vi "Haptic Master UDP.vi"() -> ()   [LabVIEW 2013]
uses:
  Common/controls/Vector3D Fingers.ctl
  labview_ros/omni_msgs/OmniFeedback.ctl
  labview_ros/geometry_msgs/Vector3.ctl
  Common/classes/MF3/MF3.lvclass
  <vilib>/Platform/TimedLoop/XDataNode/timing_clust.ctl
  <vilib>/Platform/TimedLoop/XDataNode/nitl_modes.ctl
  <vilib>/Platform/TimedLoop/XDataNode/wakeup.ctl
  labview_ros/geometry_msgs/Pose.ctl
  labview_ros/geometry_msgs/Point.ctl
  labview_ros/geometry_msgs/Quaternion.ctl
  labview_ros/omni_msgs/OmniState.ctl
  labview_ros/std_msgs/Header.ctl
  <userlib>/_matio/level5/Public/Write/Append Data Element.llb/Append Data Element (1D Array of Double).vi
  <userlib>/_matio/level5/Public/Write/Append Data Element.llb/Append Data Element (2D Array of Double).vi
  <vilib>/Platform/TimedLoop/XDataNode/XDataNode.xnode
  <userlib>/_matio/level5.lvlib
  <vilib>/Platform/TimedLoop/XDataNode/XDNodeRunTimeDep.lvlib
panel:
  out "OmniFeedback":T1
  out "Finger Positions":T3
  out "UDP Receiver":cluster{"Rate (Hz)":dbl, "Status":errorcluster}
  out "UDP Sender":cluster{"Rate (Hz)":dbl, "Status":errorcluster}
  in  "ROS Machine":T4={"IP"="192.168.0.10", "Read Port"=5053, "Write Port"=5054}
  in  "MasterFinger":T5={"PID Gains"={"Proportional Gain"=20, "Integral Gain"=5, "Derivative Gain"=0}, "Current limit"=0.0} {"Current limit" min=0.0 max=1.0 step=0.1}
  in  "Data Logging":cluster{"Path":path, "Save":bool}={"Path"=path "c:/ni-rt/testing/haptic_master.mat", "Save"=FALSE}
  out "Logging Status":errorcluster
  out "MasterFinger Status":errorcluster
  in  "Stop":bool
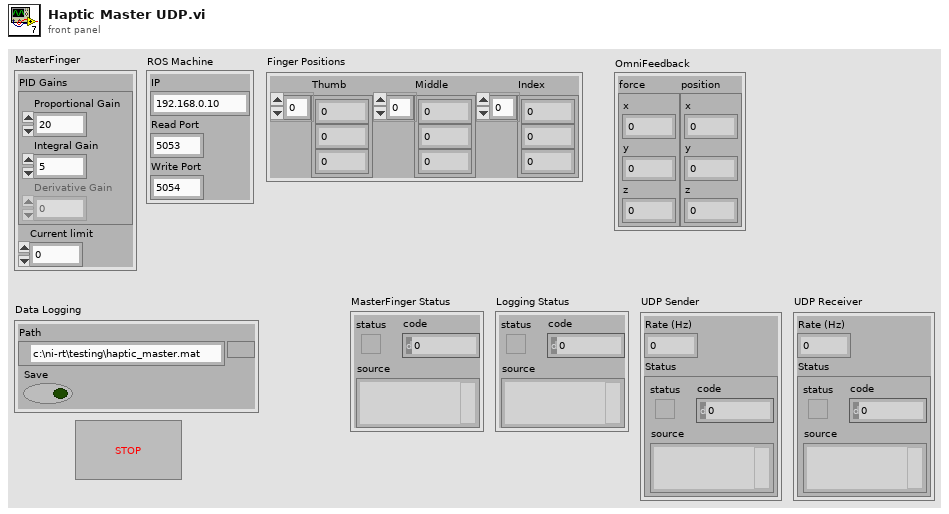
[diagram p1: front panel]
types:
  T1 = typedef "OmniFeedback.ctl" = cluster{"force":T2, "position":T2}
  T2 = typedef "Vector3.ctl" = cluster{"x":dbl, "y":dbl, "z":dbl}
  T3 = typedef "Vector3D Fingers.ctl" = cluster{"Thumb":dbl[], "Middle":dbl[], "Index":dbl[]}
  T4 = cluster{"IP":string, "Read Port":u16, "Write Port":u16}
  T5 = cluster{"PID Gains":cluster{"Proportional Gain":i16, "Integral Gain":i16, "Derivative Gain":i16}, "Current limit":dbl}
  T6 = typedef "Pose.ctl" = cluster{"position":T7, "orientation":T8}
  T7 = typedef "Point.ctl" = cluster{"x":dbl, "y":dbl, "z":dbl}
  T8 = typedef "Quaternion.ctl" = cluster{"x":dbl, "y":dbl, "z":dbl, "w":dbl}
  T9 = cluster{"Proportional Gain":i16, "Integral Gain":i16, "Derivative Gain":i16}
  T10 = typedef "XDNodeRunTimeDep.lvlib/timing_clust.ctl" = cluster{"Expected End [f-1]":u64, "Actual End [f-1]":u64, "Finished Late? [f-1]":bool, "Expected End [i-1]":u64, "Actual End [i-1]":u64, "Finished Late? [i-1]":bool, "Expected Start [i]":u64, "Actual Start [i]":u64, "Expected Start [f]":u64, "Actual Start [f]":u64, "Source Name":string, "Structure Name":string, "Period":i64, "Deadline":i64, "Offset":i64, "Start":i64, "Priority":i32, "Timeout":i32, "Mode":T11, "Wakeup Reason":T12, "Error":errorcluster, "Source Type":string, "Secondary Source Type":string, "Global End Time":u64, "Global Start Time":u64, "Frame Duration":u64, "Iteration Duration":u64, "Assigned CPU":i32, "I/O Scan Engine Mode":u32}
  T11 = typedef "XDNodeRunTimeDep.lvlib/nitl_modes.ctl" = enum32{"No Change", "Process missed periods, maintain original phase", "Discard missed periods, maintain original phase", "Process missed periods, ignore original phase", "Discard missed periods, ignore original phase"}
  T12 = typedef "XDNodeRunTimeDep.lvlib/wakeup.ctl" = enum32{"Normal", "Aborted", "Asynchronous wakeup", "Timing source error", "Timed loop error", "Timeout"}
  T13 = enum16{"big-endian, network order", "native, host order", "little-endian"}
  T14 = typedef "OmniState.ctl" = cluster{"header":T15, "locked":bool, "close_gripper":bool, "pose":T6, "current":T2, "velocity":T2}
  T15 = typedef "Header.ctl" = cluster{"seq":u32, "stamp":cluster{"sec":i32, "nsec":i32}, "frame_id":string}
  T16 = enum16{"open", "replace", "create", "open or create", "replace or create", "replace or create with confirmation"}
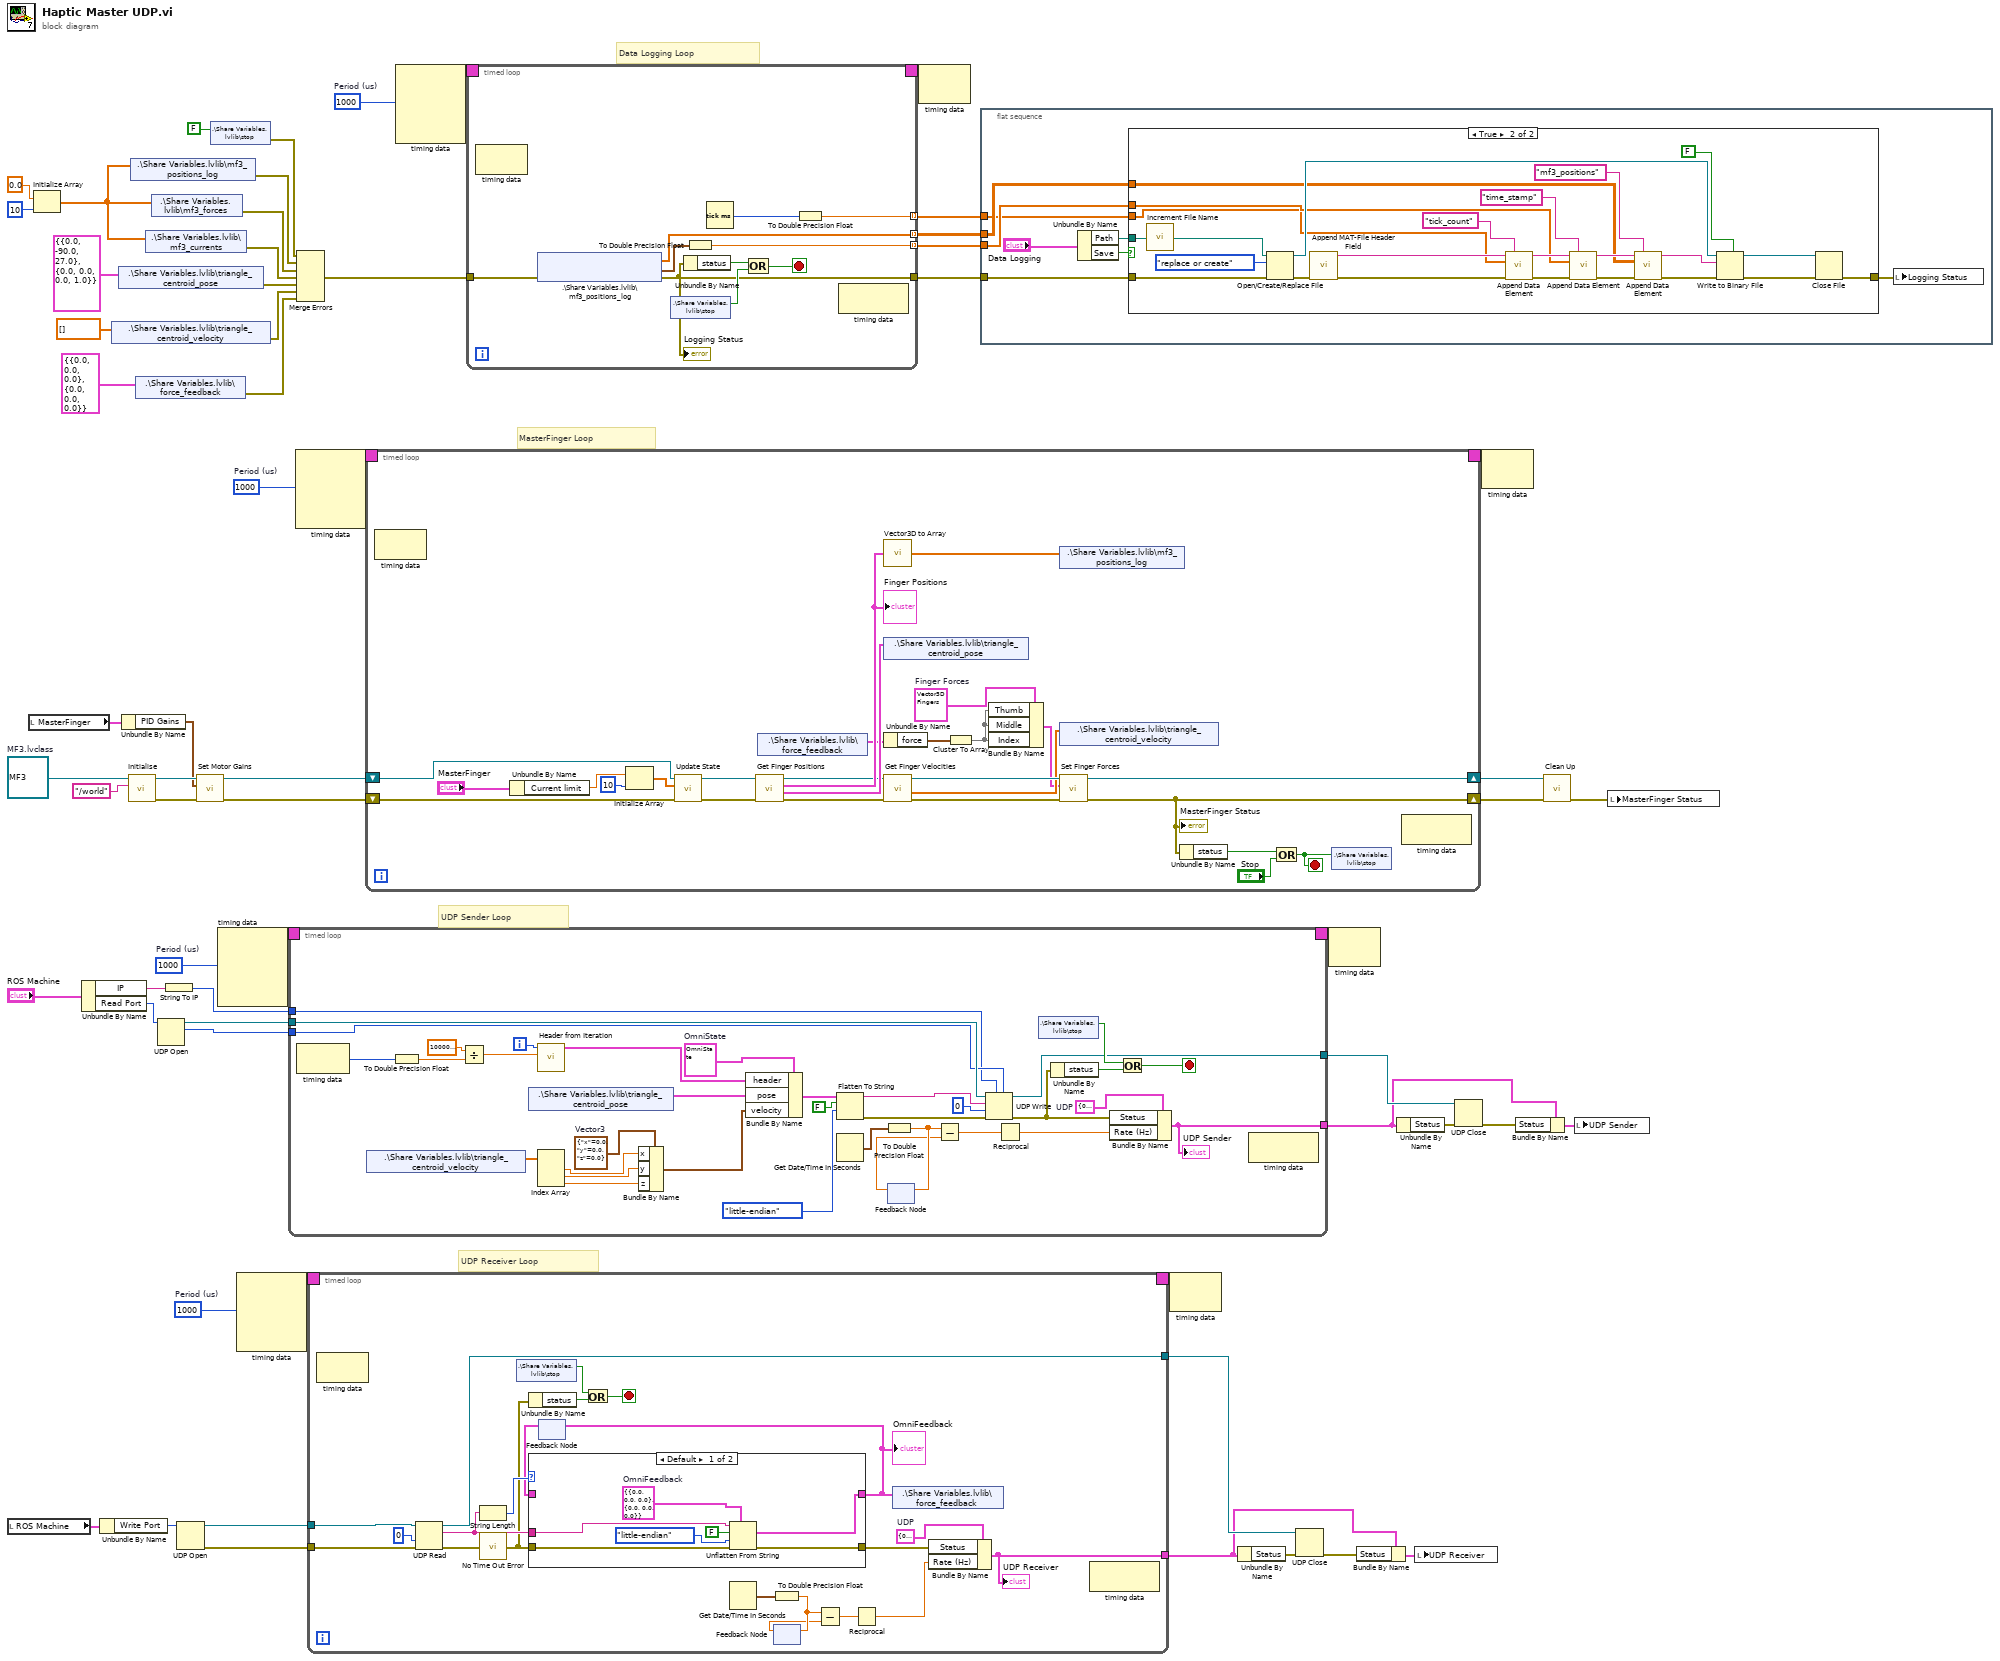
[diagram p0: block diagram]
diagram:
  w27 = i64 1000  # Period (us)
  w30 = i64 1000  # Period (us)
  w33 = i64 1000  # Period (us)
  w34 = i64 1000  # Period (us)
  w62 = refnum<class "MF3.lvclass"> refnum  # MF3.lvclass
  # "UDP Receiver Loop"
  # "UDP Sender Loop"
  # "Data Logging Loop"
  # "MasterFinger Loop"
  n1 = local read "ROS Machine"() -> (w23:T4)
  n2 = local read "MasterFinger"() -> (w44:T5)
  n3 = Initialize Array "Initialize Array"(0.0 ("element"), 10 ("dimension size")) -> (w41:dbl[])
  n4 = Unbundle By Name("ROS Machine") -> ("IP"=w26:string, "Read Port"=w24:u16)
  n5 = Unbundle By Name(w23) -> ("Write Port"=w22:u16)
  n6 = shared-variable ".\\Share Variables.lvlib\\triangle_centroid_velocity"(dbl[] [] ("triangle_centroid_velocity")) -> (error out=w4:errorcluster)  [unwired: 1 in]
  n7 = shared-variable ".\\Share Variables.lvlib\\triangle_centroid_pose"(T6 {"position"={"x"=0.0, "y"=-90.0, "z"=27.0}, "orientation"={"x"=0.0, "y"=0.0, "z"=0.0, "w"=1.0}} ("triangle_centroid_pose")) -> (error out=w6:errorcluster)  [unwired: 1 in]
  n8 = Unbundle By Name(w44) -> ("PID Gains"=w43:T9)
  n9 = call "Initialise.vi"("frame"="/world", "MF3 in"=w62) -> ("error out"=w45:errorcluster, "MF3 out"=w46:refnum<class "MF3.lvclass">)  [unwired: 8 in]
  n10 = shared-variable ".\\Share Variables.lvlib\\mf3_positions_log"(w41) -> (error out=w57:errorcluster)  [unwired: 1 in]
  n11 = shared-variable ".\\Share Variables.lvlib\\force_feedback"(T1 {"force"={"x"=0.0, "y"=0.0, "z"=0.0}, "position"={"x"=0.0, "y"=0.0, "z"=0.0}} ("force_feedback")) -> (error out=w1:errorcluster)  [unwired: 1 in]
  n12 = shared-variable ".\\Share Variables.lvlib\\mf3_currents"(w41) -> (error out=w55:errorcluster)  [unwired: 1 in]
  n13 = shared-variable ".\\Share Variables.lvlib\\mf3_forces"(w41) -> (error out=w56:errorcluster)  [unwired: 1 in]
  n14 = UDP Open(11:w24) -> (port=w21:refnum<k16>, 2:w20:u16)  [unwired: 1 in, 4 out]
  n15 = String To IP(1:w26) -> (0:w19:u32)
  n16 = UDP Open(11:w22) -> (port=w10:refnum<k16>, 0:w13:errorcluster)  [unwired: 1 in, 4 out]
  n17 = call "Set Motor Gains.vi"("error in (no error)"=w45, "motor gains"=w43, "MF3 in"=w46) -> ("error out"=w35:errorcluster, "MF3 out"=w36:refnum<class "MF3.lvclass">)  [unwired: 7 in]
  n18 = shared-variable ".\\Share Variables.lvlib\\stop"(FALSE ("stop")) -> (error out=w58:errorcluster)  [unwired: 1 in]
  n19 = node-c288(w30) -> (w32:T10)  [unwired: 3 in]
  n20 = node-c288(w27) -> (w29:T10)  [unwired: 3 in]
  n21 = timed-loop {
    timing: w32 -> [_]
    timing-out: [_] -> w31
    tunnel: w21 -> [w88]
    tunnel: w20 -> [w87]
    tunnel: w19 -> [w86]
    tunnel: [w76] -> w18
    tunnel: [w74] -> w15
    i -> [w77]
    stop <- w81 stop-if-true
    w73 = T2 {"x"=0.0, "y"=0.0, "z"=0.0}  # Vector3
    w80 = T14 {"header"={"seq"=0, "stamp"={"sec"=0, "nsec"=0}, "frame_id"=""}, "locked"=FALSE, "close_gripper"=FALSE, "pose"={"position"={"x"=0.0, "y"=0.0, "z"=0.0}, "orientation"={"x"=0.0, "y"=0.0, "z"=0.0, "w"=0.0}}, "current"={"x"=0.0, "y"=0.0, "z"=0.0}, "velocity"={"x"=0.0, "y"=0.0, "z"=0.0}}  # OmniState
    w75 = cluster{"Rate (Hz)":dbl, "Status":errorcluster} {"Rate (Hz)"=0.0, "Status"={"status"=FALSE, "code"=0, "source"=""}}  # UDP
    n22 = node-c288() -> (w66:i64)  [unwired: 1 in]
    n23 = shared-variable ".\\Share Variables.lvlib\\triangle_centroid_velocity"() -> (w72:dbl[])  [unwired: 1 in, 1 out]
    n24 = To Double Precision Float(number=w66) -> (double precision float=w65:dbl)
    n25 = Divide(x=1000000.0, y=w65) -> (x/y=w63:dbl)
    n26 = shared-variable ".\\Share Variables.lvlib\\triangle_centroid_pose"() -> (w67:T6)  [unwired: 1 in, 1 out]
    n27 = call "Header from Iteration.vi"("Rate (Hz)"=w63, "Iteration"=w77) -> ("Header"=w78:T15)  [unwired: 9 in]
    n28 = Index Array(array=w72) -> (element #1=w71:dbl, element #2=w70:dbl, element #3=w69:dbl)  [unwired: 3 in]
    n29 = Bundle By Name(cluster=w73, "x"=w71, "y"=w70, "z"=w69) -> (w68:T2)
    n30 = Bundle By Name(cluster=w80, "header"=w78, "pose"=w67, "velocity"=w68) -> (w79:T14)
    n31 = Flatten To String(anything=w79, prepend array or string size? (T)=FALSE, byte order (0:big-endian, network order)=T13."little-endian") -> (data string=w89:string, error out=w85:errorcluster)  [unwired: 1 in, 1 out]
    n32 = Get Date/Time In Seconds() -> (seconds since 1Jan1904=w94:timestamp)
    n33 = To Double Precision Float(number=w94) -> (double precision float=w92:dbl)
    n34 = feedback #1() -> (w91:dbl)  [unwired: 1 in]
    n35 = feedback-in #1(w92) -> ()
    n36 = Subtract(x=w92, y=w91) -> (x-y=w95:dbl)
    n37 = UDP Write(address=w86, port or service name=w87, connection ID=w88, data in=w89, 8:w85, 9:0 ("timeout ms (25000)")) -> (error out=w84:errorcluster, 3:w76:refnum<k16>)
    n38 = Reciprocal(x=w95) -> (1/x=w93:dbl)
    n39 = shared-variable ".\\Share Variables.lvlib\\stop"() -> (w83:bool)  [unwired: 1 in, 1 out]
    n40 = Unbundle By Name(w84) -> ("status"=w82:bool)
    n41 = Bundle By Name(cluster=w75, "Status"=w84, "Rate (Hz)"=w93) -> (w74:cluster{"Rate (Hz)":dbl, "Status":errorcluster})
    "UDP Sender" <- w74
    n42 = Or(x=w83, y=w82) -> (x .or. y?=w81:bool)
    n43 = node-c288() -> ()  [unwired: 1 in, 1 out]
  }
  n44 = node-c288(w34) -> (w40:T10)  [unwired: 3 in]
  n45 = Merge Errors(w58, w57, w56, w55, w6, w4, w1) -> (w48:errorcluster)
  n46 = timed-loop {
    timing: w29 -> [_]
    timing-out: [_] -> w28
    tunnel: w13 -> [w112]
    tunnel: w10 -> [w111]
    tunnel: [w110] -> w9
    tunnel: [w115] -> w8
    stop <- w107 stop-if-true
    w116 = cluster{"Rate (Hz)":dbl, "Status":errorcluster} {"Rate (Hz)"=0.0, "Status"={"status"=FALSE, "code"=0, "source"=""}}  # UDP
    n47 = node-c288() -> ()  [unwired: 1 in, 1 out]
    n48 = UDP Read(connection ID=w111, timeout ms (25000)=0 ("timeout (ms)"), 8:w112) -> (data out=w105:string, error out=w114:errorcluster, 3:w110:refnum<k16>)  [unwired: 1 in, 2 out]
    n49 = String Length(string=w105) -> (length=w106:i32)
    n50 = call <vilib>:"No Time Out Error.vi"("error in (no error)"=w114) -> ("error out"=w104:errorcluster)  [unwired: 14 out]
    n51 = shared-variable ".\\Share Variables.lvlib\\stop"() -> (w108:bool)  [unwired: 1 in, 1 out]
    n52 = Unbundle By Name(w104) -> ("status"=w109:bool)
    n53 = feedback #2() -> (w103:T1)  [unwired: 1 in]
    n54 = case shown="Default" w106 {
      tunnel: w104 -> [w123 w130]
      tunnel: [w127 w130] -> w102
      tunnel: [w125 w129] -> w101
      tunnel: w105 -> [w124 _]
      tunnel: w103 -> [_ w129]
      frame Default {
        w122 = T1 {"force"={"x"=0.0, "y"=0.0, "z"=0.0}, "position"={"x"=0.0, "y"=0.0, "z"=0.0}}  # OmniFeedback
        n55 = Unflatten From String(type=w122, binary string=w124, data includes array or string size? (T)=FALSE, byte order (0:big-endian, network order)=T13."little-endian", error in (no error)=w123) -> (value=w125:T1, error out=w127:errorcluster)  [unwired: 1 out]
      }
      frame 0 {
      }
    }
    "OmniFeedback" <- w101
    n56 = feedback-in #2(w101) -> ()
    n57 = Or(x=w108, y=w109) -> (x .or. y?=w107:bool)
    n58 = Get Date/Time In Seconds() -> (seconds since 1Jan1904=w120:timestamp)
    n59 = To Double Precision Float(number=w120) -> (double precision float=w118:dbl)
    n60 = feedback #3() -> (w117:dbl)  [unwired: 1 in]
    n61 = feedback-in #3(w118) -> ()
    n62 = Subtract(x=w118, y=w117) -> (x-y=w121:dbl)
    n63 = Reciprocal(x=w121) -> (1/x=w119:dbl)
    n64 = shared-variable ".\\Share Variables.lvlib\\force_feedback"(w101) -> ()  [unwired: 1 in, 1 out]
    n65 = Bundle By Name(cluster=w116, "Status"=w102, "Rate (Hz)"=w119) -> (w115:cluster{"Rate (Hz)":dbl, "Status":errorcluster})
    "UDP Receiver" <- w115
    n66 = node-c288() -> ()  [unwired: 1 in, 1 out]
  }
  n67 = timed-loop {
    shift-right: [w147] -> w60
    shift-left: w36 -> [w150]
    shift-right: [w146] -> w54
    shift-left: w35 -> [w149]
    timing: w40 -> [_]
    timing-out: [_] -> w39
    stop <- w153 stop-if-true
    w139 = T3 {"Thumb"=[0.0, 0.0, 0.0], "Middle"=[0.0, 0.0, 0.0], "Index"=[0.0, 0.0, 0.0]}  # Finger Forces
    n68 = node-c288() -> ()  [unwired: 1 in, 1 out]
    n69 = Unbundle By Name("MasterFinger") -> ("Current limit"=w156:dbl)
    n70 = Initialize Array(w156, 10 ("dimension size")) -> (w154:dbl[])
    n71 = call "Update State.vi"("error in (no error)"=w149, "current_limits"=w154, "MF3 in"=w150) -> ("error out"=w133:errorcluster, "MF3 out"=w134:refnum<class "MF3.lvclass">)  [unwired: 7 in]
    n72 = call "Get Finger Positions.vi"("error in (no error)"=w133, "MF3 in"=w134) -> ("error out"=w141:errorcluster, "Triangle Centroid Pose"=w145:T6, "Finger Positions"=w151:T3, "MF3 out"=w144:refnum<class "MF3.lvclass">)  [unwired: 6 in]
    "Finger Positions" <- w151
    n73 = shared-variable ".\\Share Variables.lvlib\\force_feedback"() -> (w138:T1)  [unwired: 1 in, 1 out]
    n74 = call "Vector3D to Array.vi"("Vector3D"=w151) -> ("Array"=w158:dbl[])
    n75 = shared-variable ".\\Share Variables.lvlib\\triangle_centroid_pose"(w145) -> ()  [unwired: 1 in, 1 out]
    n76 = Unbundle By Name(w138) -> ("force"=w136:T2)
    n77 = call "Get Finger Velocities.vi"("error in (no error)"=w141, "MF3 in"=w144) -> ("error out"=w142:errorcluster, "Triangle Centroid Velocity"=w140:dbl[], "MF3 out"=w143:refnum<class "MF3.lvclass">)  [unwired: 6 in, 1 out]
    n78 = Cluster To Array(cluster=w136) -> (array=w135:dbl[])
    n79 = Bundle By Name(cluster=w139, "Thumb"=w135, "Middle"=w135, "Index"=w135) -> (w137:T3)
    n80 = shared-variable ".\\Share Variables.lvlib\\mf3_positions_log"(w158) -> ()  [unwired: 1 in, 1 out]
    n81 = shared-variable ".\\Share Variables.lvlib\\triangle_centroid_velocity"(w140) -> ()  [unwired: 1 in, 1 out]
    n82 = call "Set Finger Forces.vi"("error in (no error)"=w142, "Finger Forces"=w137, "MF3 in"=w143) -> ("error out"=w146:errorcluster, "MF3 out"=w147:refnum<class "MF3.lvclass">)  [unwired: 6 in, 1 out]
    "MasterFinger Status" <- w146
    n83 = Unbundle By Name(w146) -> ("status"=w148:bool)
    n84 = Compound Arithmetic op=OR(w148, "Stop") -> (w153:bool)
    n85 = shared-variable ".\\Share Variables.lvlib\\stop"(w153) -> ()  [unwired: 1 in, 1 out]
    n86 = node-c288() -> ()  [unwired: 1 in, 1 out]
  }
  n87 = node-c288(w33) -> (w38:T10)  [unwired: 3 in]
  n88 = timed-loop {
    tunnel: [w166] -> w47
    tunnel: w48 -> [w170]
    tunnel: [w163] -> w51 mode=indexing
    tunnel: [w162] -> w50 mode=indexing
    tunnel: [w161] -> w49 mode=indexing
    timing: w38 -> [_]
    timing-out: [_] -> w37
    stop <- w167 stop-if-true
    n89 = node-c288() -> ()  [unwired: 1 in, 1 out]
    n90 = shared-variable ".\\Share Variables.lvlib\\mf3_positions_log"(error in=w170) -> (w163:dbl[], error out=w166:errorcluster, w164:timestamp)
    "Logging Status" <- w166
    n91 = shared-variable ".\\Share Variables.lvlib\\stop"() -> (w169:bool)  [unwired: 1 in, 1 out]
    n92 = Unbundle By Name(w166) -> ("status"=w168:bool)
    n93 = To Double Precision Float(number=w164) -> (double precision float=w162:dbl)
    n94 = Tick Count (ms)() -> (millisecond timer value=w165:u32)
    n95 = Compound Arithmetic op=OR(w168, w169) -> (w167:bool)
    n96 = To Double Precision Float(number=w165) -> (double precision float=w161:dbl)
    n97 = node-c288() -> ()  [unwired: 1 in, 1 out]
  }
  n98 = node-c288(w37) -> ()  [unwired: 1 out]
  n99 = flat-sequence {
    tunnel: w51 -> [w179]
    tunnel: w50 -> [w178]
    tunnel: w49 -> [w177]
    tunnel: w47 -> [w176]
    frame #0 {
      n100 = Unbundle By Name("Data Logging") -> ("Path"=w174:path, "Save"=w173:bool)
      n101 = case shown="True" w173 {
        tunnel: [w181 w190] -> w180
        tunnel: w179 -> [_ w189]
        tunnel: w178 -> [_ w188]
        tunnel: w177 -> [_ w187]
        tunnel: w176 -> [w181 w186]
        tunnel: w174 -> [_ w184]
        frame False {
        }
        frame True {
          n102 = call "Increment File Name.vi"("Full Path"=w184) -> ("New Path"=w191:path)
          n103 = Open/Create/Replace File(file path (use dialog)=w191, error in=w186, operation (0:open)=T16."replace or create") -> (refnum out=w192:refnum<file>, error out=w185:errorcluster)  [unwired: 3 in, 1 out]
          n104 = call <userlib>:"Append MAT-File Header Field.vi"("error"=w185) -> ("result string"=w201:string, "error out"=w200:errorcluster)  [unwired: 13 in]
          n105 = call-poly <userlib>:"Append Data Element.vi"("initial string"=w201, "Data Name"="tick_count", "data"=w187, "error in"=w200) -> ("result string"=w195:string, "error out"=w194:errorcluster)  [unwired: 10 in]
          n106 = call-poly <userlib>:"Append Data Element.vi"("initial string"=w195, "Data Name"="time_stamp", "data"=w188, "error in"=w194) -> ("result string"=w197:string, "error out"=w196:errorcluster)  [unwired: 10 in]
          n107 = call-poly <userlib>:"Append Data Element.vi"("initial string"=w197, "Data Name"="mf3_positions" ("array name"), "data"=w189, "error in"=w196) -> ("result string"=w183:string, "error out"=w182:errorcluster)  [unwired: 10 in]
          n108 = Write to Binary File(file (use dialog)=w192, data=w183, error in=w182, 5:FALSE ("prepend array or string size? (T)")) -> (refnum out=w203:refnum<file>, error out=w202:errorcluster)  [unwired: 2 in, 1 out]
          n109 = Close File(refnum=w203, error in=w202) -> (error out=w190:errorcluster)  [unwired: 1 out]
        }
      }
      n110 = local write "Logging Status"(w180) -> ()
    }
  }
  n111 = node-c288(w28) -> ()  [unwired: 1 out]
  n112 = Unbundle By Name(w8) -> ("Status"=w12:errorcluster)
  n113 = UDP Close(connection ID=w9, 8:w12) -> (error out=w11:errorcluster)  [unwired: 1 out]
  n114 = node-c288(w31) -> ()  [unwired: 1 out]
  n115 = Bundle By Name(cluster=w8, "Status"=w11) -> (w7:cluster{"Rate (Hz)":dbl, "Status":errorcluster})
  n116 = Unbundle By Name(w15) -> ("Status"=w17:errorcluster)
  n117 = local write "UDP Receiver"(w7) -> ()
  n118 = UDP Close(connection ID=w18, 8:w17) -> (error out=w16:errorcluster)  [unwired: 1 out]
  n119 = node-c288(w39) -> ()  [unwired: 1 out]
  n120 = Bundle By Name(cluster=w15, "Status"=w16) -> (w14:cluster{"Rate (Hz)":dbl, "Status":errorcluster})
  n121 = call "Clean Up.vi"("error in (no error)"=w54, "MF3 in"=w60) -> ("error out"=w42:errorcluster)  [unwired: 8 in, 1 out]
  n122 = local write "UDP Sender"(w14) -> ()
  n123 = local write "MasterFinger Status"(w42) -> ()
